vi "PrepareSequenceAcquisition.vi"(8 "error in (no error)":errorcluster, 11 "Camera_Prime95B in":refnum<class "Camera_Prime95B.lvclass">) -> (0 "error out":errorcluster, 3 "Camera_Prime95B out":refnum<class "Camera_Prime95B.lvclass">)   [LabVIEW 2020, in "Camera_Prime95B.lvlib" / "Camera_Prime95B.lvclass"]
uses:
  Camera_Prime95B.lvclass
  Camera_Prime95B.lvclass/Camera_Prime95B.ctl
  E:/Development/DevHardSoftware/MicroscopyFramework/Model/Hardware Layer/Real Hardware/Camera_Prime95B/Camera_Prime95B/Dependencies/PVCamNET.dll
  Dependencies/PVCamNET.dll
  Hardware Abstraction Layer/Component/Camera/Camera/Camera.lvclass
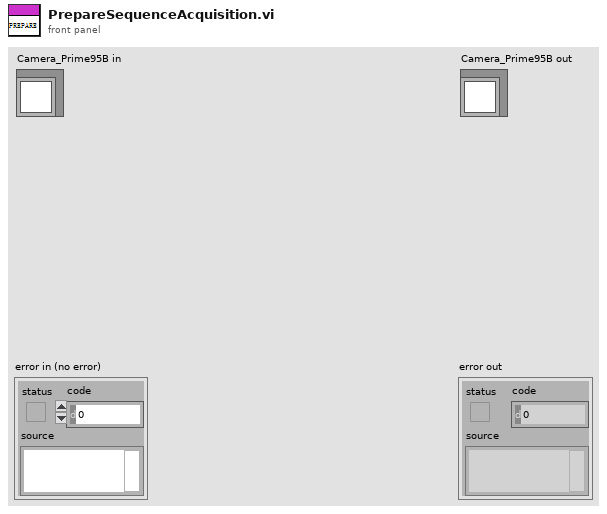
[diagram p1: front panel]
types:
  T1 = typedef "Device.lvlib/DeviceStatus.ctl" = i32
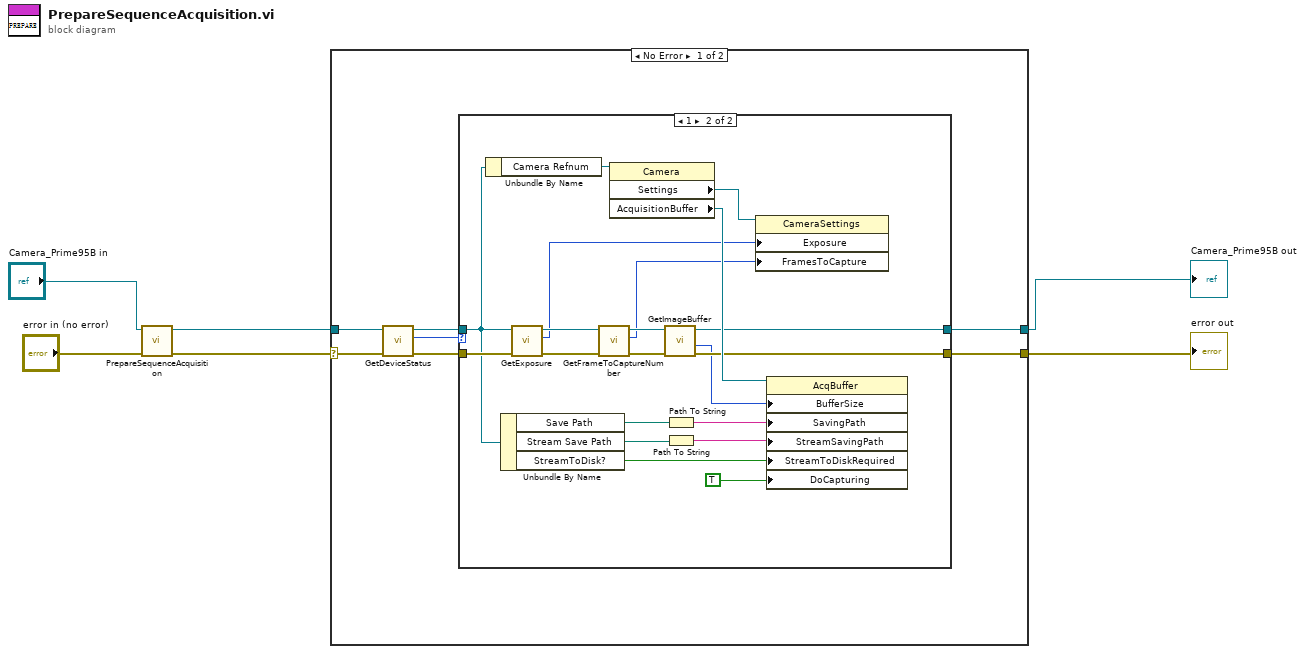
[diagram p0: block diagram]
diagram:
  n1 = call-parent "PrepareSequenceAcquisition.vi"("error in (no error)"="error in (no error)", "Device in"="Camera_Prime95B in") -> ("error out"=w4:errorcluster, "Device out"=w2:refnum<class "Camera_Prime95B.lvclass">)  [unwired: 8 in]
  n2 = case shown="No Error" w4 {
    selector: w4 -> [w13 w37]
    tunnel: [w11 w37] -> w3
    tunnel: w2 -> [w9 w36]
    tunnel: [w12 w36] -> w1
    frame No Error {
      n3 = call-dynamic "GetDeviceStatus.vi"("error in (no error)"=w13, "Camera_Prime95B in"=w9) -> ("error out"=w10:errorcluster, "Status"=w7:T1, "Camera_Prime95B out"=w8:refnum<class "Camera_Prime95B.lvclass">)  [unwired: 7 in]
      n4 = case shown="1" w7 {
        tunnel: w8 -> [w15 w20]
        tunnel: w10 -> [w14 w27]
        tunnel: [w15 w21] -> w12
        tunnel: [w14 w23] -> w11
        frame 0, Default {
        }
        frame 1 {
          n5 = Unbundle By Name(w20) -> ("Camera Refnum"=w35:refnum<k24>)
          n6 = Unbundle By Name(w20) -> ("Save Path"=w32:path, "Stream Save Path"=w31:path, "StreamToDisk?"=w29:bool)
          n7 = call-dynamic "GetExposure.vi"("error in (no error)"=w27, "Camera in"=w20) -> ("error out"=w26:errorcluster, "Setting.Exposure"=w19:i32, "Camera out"=w24:refnum<class "Camera_Prime95B.lvclass">)  [unwired: 7 in]
          n8 = call-dynamic "GetFrameToCaptureNumber.vi"("error in (no error)"=w26, "Camera in"=w24) -> ("error out"=w25:errorcluster, "Setting.FramesToCapture"=w18:i32, "Camera out"=w22:refnum<class "Camera_Prime95B.lvclass">)  [unwired: 7 in]
          n9 = property class="Camera"(reference=w35) -> ("Settings"=w34:refnum<k24>, "AcquisitionBuffer"=w33:refnum<k24>)  [unwired: 1 in, 2 out]
          n10 = call-dynamic "GetImageBuffer.vi"("error in (no error)"=w25, "Camera in"=w22) -> ("error out"=w23:errorcluster, "Setting.BufferSize"=w16:i32, "Camera out"=w21:refnum<class "Camera_Prime95B.lvclass">)  [unwired: 6 in, 1 out]
          n11 = Path To String(path=w32) -> (string=w17:string)
          n12 = Path To String(path=w31) -> (string=w30:string)
          n13 = property class="CameraSettings"(reference=w34, "Exposure"=w19, "FramesToCapture"=w18) -> ()  [unwired: 1 in, 2 out]
          n14 = property class="AcqBuffer"(reference=w33, "BufferSize"=w16, "SavingPath"=w17, "StreamSavingPath"=w30, "StreamToDiskRequired"=w29, "DoCapturing"=TRUE) -> ()  [unwired: 1 in, 2 out]
        }
      }
    }
    frame Error {
    }
  }
  "error out" <- w3
  "Camera_Prime95B out" <- w1
